vi "Fetch Multi Eval Meas SEM Margin Results.vi"(6 "Offset Frequency (Positive)":i32(ring)=1 items=["Negative", "Positive"], 8 "error in (no error)":errorcluster, 9 "Result Type (Current)":i32(ring) items=["Current"=0, "Average"=1, "Minimum"=5], 10 "Instance (1)":T1=1, 11 "VISA resource name":refnum<visa-resource-name>) -> (0 "error out":errorcluster, 1 "SEM Margin Results":cluster{"Margin X":dbl, "Margin Y":dbl}[](array[cluster]) {"Margin Y" format="%^.3e"; "Margin X" format="%^.3e"}, 2 "Reliability":i32, 3 "VISA resource name out":refnum<visa-resource-name>, 5 "Out Of Tolerance":i32)   [LabVIEW 2020, in "Rohde&Schwarz CMWXP NR FR1 Measurement.lvlib"]
doc: "Returns spectrum emission mask margin results. A negative margin indicates that the trace is located above the limit line, i.e. the limit is exceeded.\n\nResults for the current, average and maximum traces (resulting in minimum margins) can be returned for negative and positive offset frequencies. For each trace, the X and Y values of the margins for emission mask areas 1 to 12 are provided. For inactive areas, NCAP is returned.\n\nAttributes:\nRSCMWXPNRFR1M_ATTR_FETCH_MULTI_EVAL_MEAS_SEM_MARGIN_POSITIVE_CURRENT_RESULTS\nRSCMWXPNRFR1M_ATTR_FETCH_MULTI_EVAL_MEAS_SEM_MARGIN_POSITIVE_AVERAGE_RESULTS\nRSCMWXPNRFR1M_ATTR_FETCH_MULTI_EVAL_MEAS_SEM_MARGIN_POSITIVE_MINIMUM_RESULTS\nRSCMWXPNRFR1M_ATTR_FETCH_MULTI_EVAL_MEAS_SEM_MARGIN_NEGATIVE_CURRENT_RESULTS\nRSCMWXPNRFR1M_ATTR_FETCH_MULTI_EVAL_MEAS_SEM_MARGIN_NEGATIVE_AVERAGE_RESULTS\nRSCMWXPNRFR1M_ATTR_FETCH_MULTI_EVAL_MEAS_SEM_MARGIN_NEGATIVE_MINIMUM_RESULTS\n\nRemote-control commands:\nFETCh:NRSub:MEAS<i>:MEValuation:SEMask:MARGin:CURRent:POSitiv?\nFETCh:NRSub:MEAS<i>:MEValuation:SEMask:MARGin:AVERage:POSitiv?\nFETCh:NRSub:MEAS<i>:MEValuation:SEMask:MARGin:MINimum:POSitiv?\nFETCh:NRSub:MEAS<i>:MEValuation:SEMask:MARGin:CURRent:NEGativ?\nFETCh:NRSub:MEAS<i>:MEValuation:SEMask:MARGin:AVERage:NEGativ?\nFETCh:NRSub:MEAS<i>:MEValuation:SEMask:MARGin:MINimum:NEGativ?"
uses:
  <instrlib>/Rohde&Schwarz CMWXP NR FR1 Measurement/Rohde&Schwarz CMWXP NR FR1 Measurement.lvlib
  <instrlib>/Rohde&Schwarz CMWXP NR FR1 Measurement/Private/_Instance.ctl
  <instrlib>/Rohde&Schwarz CMWXP NR FR1 Measurement/Private/rsidr_core.llb/rsidr_core.lvlib
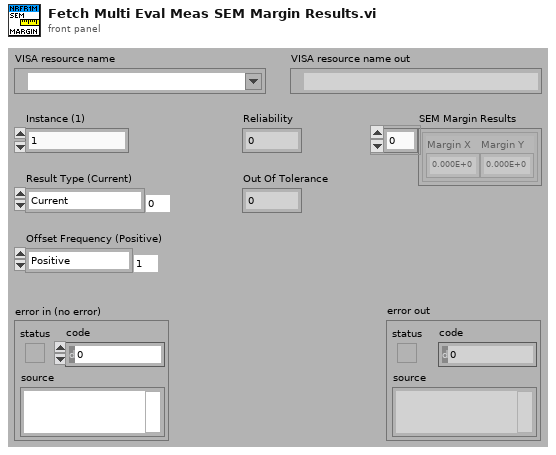
[diagram p1: front panel]
types:
  T1 = typedef "Rohde&Schwarz CMWXP NR FR1 Measurement.lvlib/_Instance.ctl" = i32
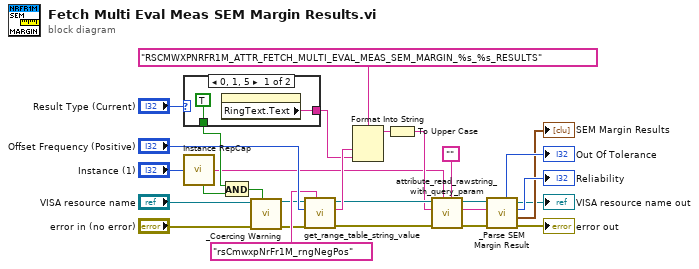
[diagram p0: block diagram]
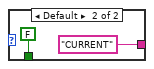
[diagram p2: hidden frame]
diagram:
  n1 = case shown="0, 1, 5" "Result Type (Current)" {
    tunnel: [w30 "CURRENT"] -> w18
    tunnel: [TRUE FALSE] -> w15
    frame 0, 1, 5 {
      n2 = property on="Result Type (Current)" class="Ring (strict)"() -> ("RingText.Text"=w30:string)  [unwired: 2 in, 2 out]
    }
    frame Default {
    }
  }
  n3 = call <instrlib>:"Instance RepCap.vi"("Instance In"="Instance (1)") -> ("In Range?"=w16:bool, "RepCap Identifier Out"=w10:string)  [unwired: 1 in]
  n4 = And(x=w15, y=w16) -> (x .and. y?=w17:bool)
  n5 = call <instrlib>:"_Coercing Warning.vi"("In Range?"=w17, "error in (no error)"="error in (no error)", "VISA resource name"="VISA resource name") -> ("error out"=w22:errorcluster, "VISA resource name out"=w23:refnum<visa-resource-name>)  [unwired: 7 in]
  n6 = call <instrlib>:"get_range_table_string_value.vi"("Range Table ID in"="rsCmwxpNrFr1M_rngNegPos", "error in"=w22, "I32 input"="Offset Frequency (Positive)", "VISA resource name"=w23) -> ("error out"=w11:errorcluster, "String Value out"=w19:string, "VISA resource name out"=w14:refnum<visa-resource-name>)  [unwired: 5 in]
  n7 = Format Into String(format string="RSCMWXPNRFR1M_ATTR_FETCH_MULTI_EVAL_MEAS_SEM_MARGIN_%s_%s_RESULTS", w19, w18) -> (resulting string=w13:string)  [unwired: 2 in, 1 out]
  n8 = To Upper Case(1:w13) -> (0:w12:string)
  n9 = call <instrlib>:"attribute_read_rawstring_with_query_param.vi"("Query Parameter (None)"="", "Repeated Capability"=w10, "error in"=w11, "Attribute ID"=w12, "VISA resource name"=w14) -> ("error out"=w8:errorcluster, "Raw String out"=w7:string, "VISA resource name out"=w6:refnum<visa-resource-name>)  [unwired: 4 in]
  n10 = call <instrlib>:"_Parse SEM Margin Result.vi"("error in (no error)"=w8, "Input String"=w7, "VISA resource name"=w6) -> ("error out"=→"error out":errorcluster, "SEM Margin Results"=→"SEM Margin Results":cluster{"Margin X":dbl, "Margin Y":dbl}[], "Reliability"=→"Reliability":i32, "VISA resource name out"=→"VISA resource name out":refnum<visa-resource-name>, "Out Of Tolerance"=→"Out Of Tolerance":i32)  [unwired: 4 in]
